vi "LISVwithout21-10-2019.vi"() -> ()   [LabVIEW 2018]
uses:
  <instrlib>/Keithley 6517/Keithley 6517.lvlib
  <instrlib>/Keithley 2450/Keithley 2450.lvlib
panel:
  out "Photodiode":cluster{dbl[], dbl[]}(graph)
  out "LED":cluster{dbl[], dbl[]}(graph)
  out "Number of times the K6514 buffer wait loop ran":i32
  in  "Measure settings":T1={"Keithley 2450 \nMeasurement speed (PLC)"=1.0, "High capacitance?"=FALSE, "Keithley 6514 \nMeasurement speed (PLC)"=0.05, "LED: number of readings to average/measurement"=10, "Photodiode: number of readings to average/measurement"=10, "OD3 engaged on 918D?"=TRUE} {"Photodiode: number of readings to average/measurement" items=["10"=10, "50"=50, "100"=100]; "LED: number of readings to average/measurement" items=["10"=10, "50"=50, "100"=100]}
  out "Number of Readings Retrieved from K6514":i32
  in  "File I/O (in strings below, use a single word, no spaces or special characters other than -)":T2={"Experiment Name"="", "LV Data folder"=path "", "Device number"=1, "Repetition Number"=1, "Extra comment"=""}
  in  "LED bias settings":T3={"Steps (number)"=51, "Vdevice (starting, V)"=0.0, "Vdevice (ending, V)"=5.0, "Accurate readback?"=TRUE, "Current compliance (A)"=0.1} {"Vdevice (ending, V)" min=0.1 max=12.0 step=0.05; "Vdevice (starting, V)" min=0.0 max=20.0 step=0.05; "Steps (number)" min=5 max=1001 step=1}
  in  "VISA Resource IDs":T4={"VISA resource name (Keithley 2450)"="TCPIP0::192.168.30.14::inst0::INSTR", "VISA resource name (Keithley 6514)"="GPIB0::16::INSTR"}
  out "error out":errorcluster
  in  "error in (no error)":errorcluster
  # "1"
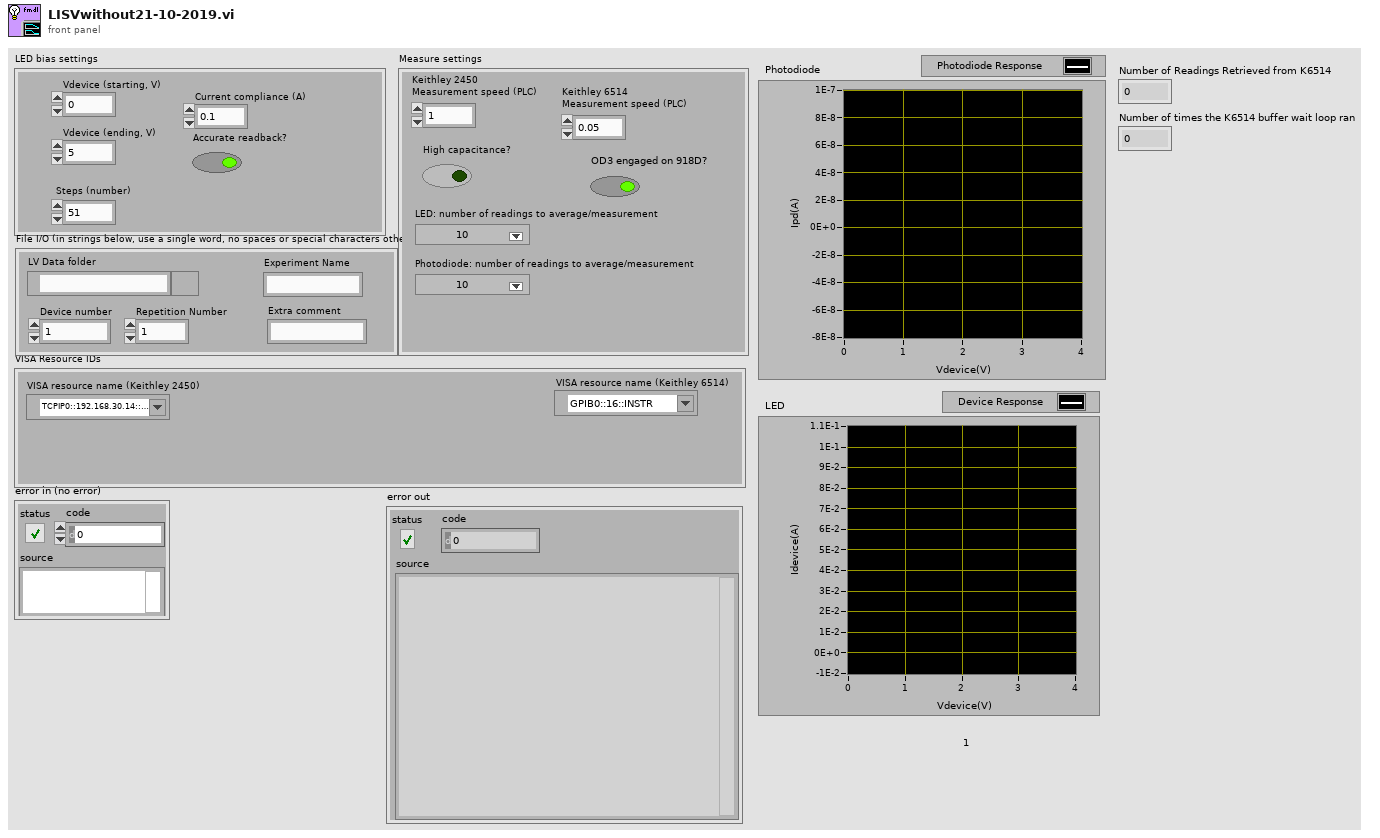
[diagram p1: front panel]
types:
  T1 = cluster{"Keithley 2450 \nMeasurement speed (PLC)":dbl, "High capacitance?":bool, "Keithley 6514 \nMeasurement speed (PLC)":dbl, "LED: number of readings to average/measurement":u16, "Photodiode: number of readings to average/measurement":u16, "OD3 engaged on 918D?":bool}
  T2 = cluster{"Experiment Name":string, "LV Data folder":path, "Device number":u32, "Repetition Number":u32, "Extra comment":string}
  T3 = cluster{"Steps (number)":i32, "Vdevice (starting, V)":dbl, "Vdevice (ending, V)":dbl, "Accurate readback?":bool, "Current compliance (A)":dbl}
  T4 = cluster{"VISA resource name (Keithley 2450)":refnum<visa-resource-name>, "VISA resource name (Keithley 6514)":refnum<visa-resource-name>}
  T5 = enum16{"open", "replace", "create", "open or create", "replace or create", "replace or create with confirmation"}
  T6 = cluster{dbl, "Mean":dbl, "StDev":dbl, "Mean":dbl, "Standard Deviation":dbl, dbl, dbl}
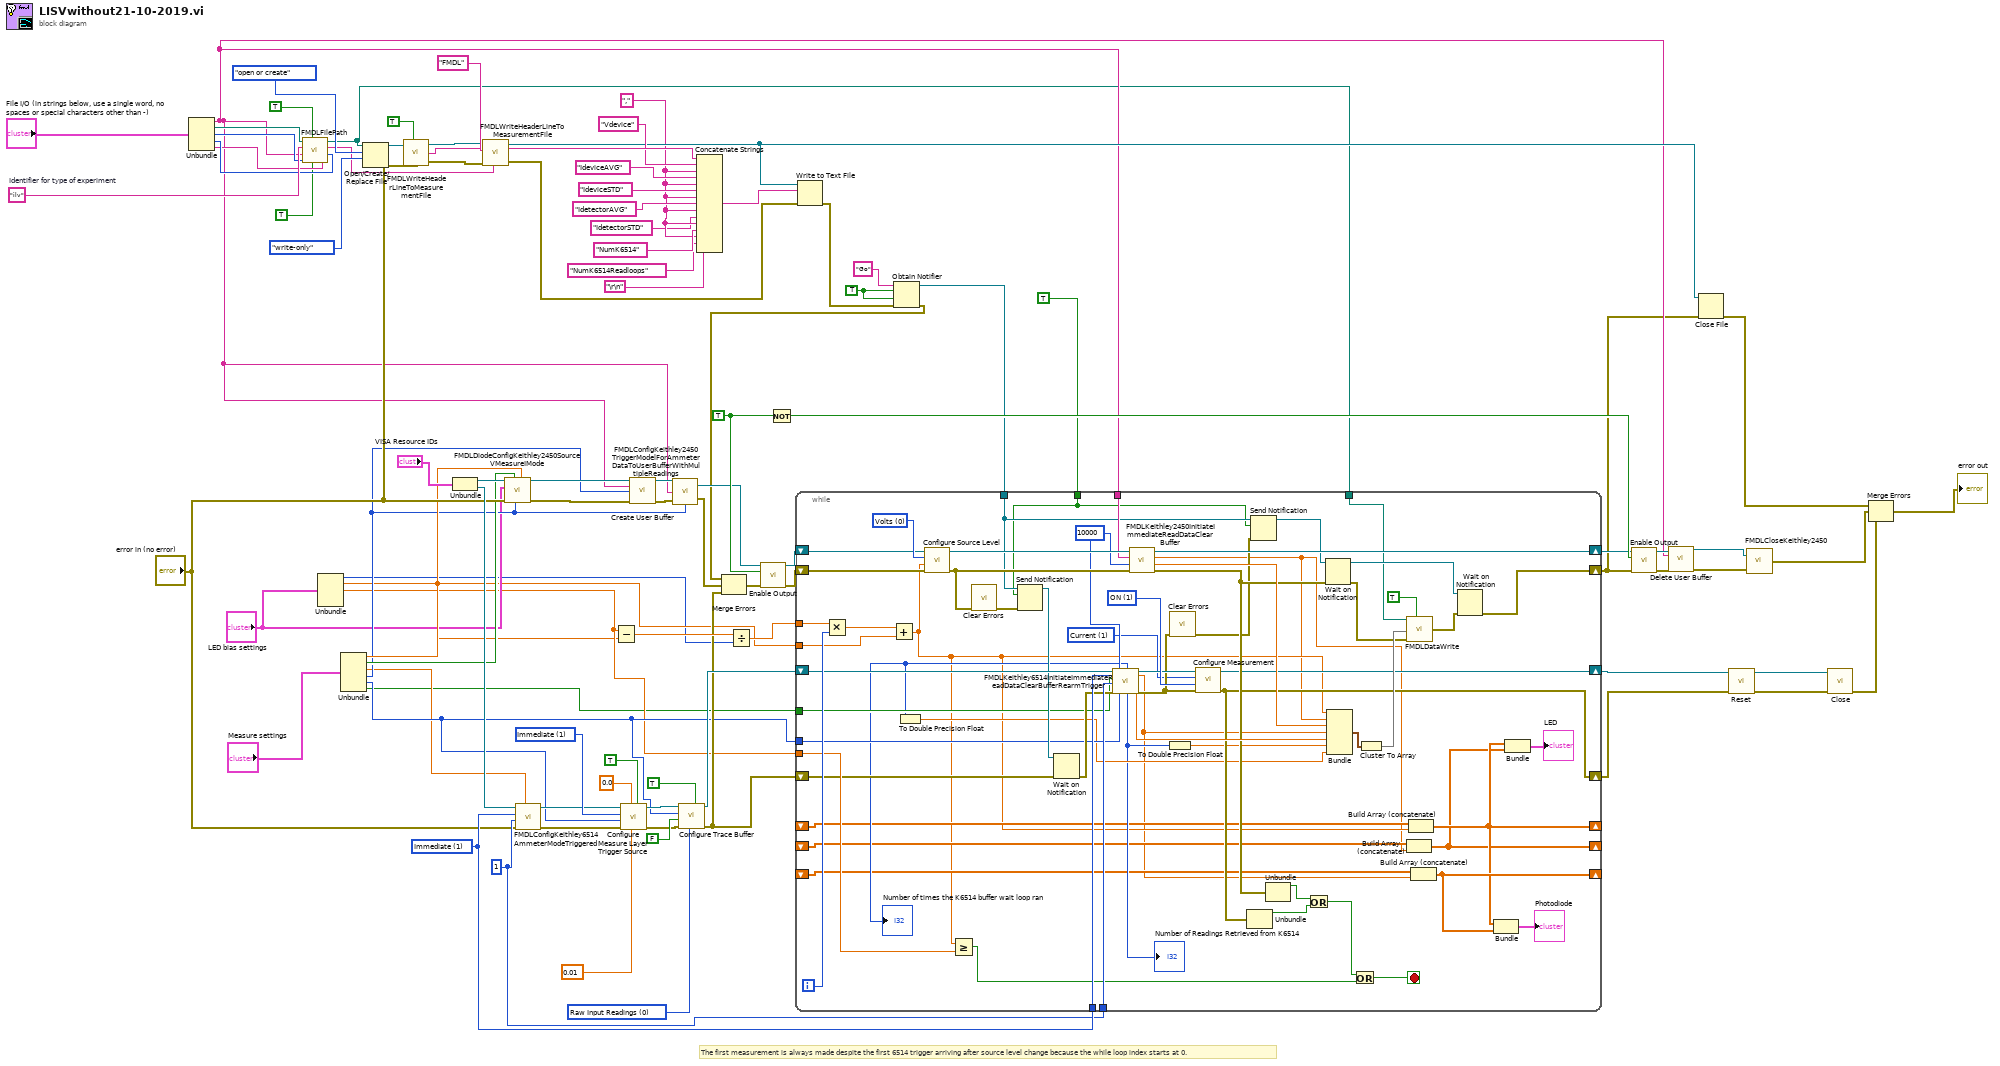
[diagram p0: block diagram]
diagram:
  w25 = TRUE ("create if not found? (T)")
  w9 = ","
  w67 = "ilv"  # Identifier for type of experiment
  w76 = 1 items=["Hold"=0, "Immediate"=1, "Manual"=3, "Bus"=4, "Trigger Link"=5, "External Triggering"=6, "Timer "=7] ("Measure Source (1: Immediate)")
  w77 = 1 ("Arm Count (1)")
  w78 = 1 items=["Hold", "Immediate", "Real-time Clock", "Manual", "Bus", "Trigger Link", "External Triggering", "Timer", "STest", "PSTest", "NSTest", "BSTest"] ("Arm Source (1: Immediate)")
  w81 = u16 0 items=["Raw Input Readings", "CALC1 Readings", "CALC2 Readings"] ("Buffer Source (0: Raw Input Readings)")
  w90 = TRUE ("Enable Output (T: Enable)")
  # "The first measurement is always made despite the first 6514 trigger arriving after source level change because the while loop index starts at 0."
  n1 = Unbundle("File I/O (in strings below, use a single word, no spaces or special characters other than -)") -> ("Experiment Name"=w36:string, "LV Data folder"=w68:path, "Device number"=w66:u32, "Repetition Number"=w65:u32, "Extra comment"=w64:string)
  n2 = call "FMDLFilePath.vi"("Extra comment"=w64, "Repetition Number"=w65, "Include seconds string?"=TRUE, "Include Year Month string?"=TRUE, "Experiment number"=w66, "Experiment Name"=w36, "Experiment Type"=w67, "Data folder"=w68) -> ("date/time string"=w52:string, "Unique Filepath"=w23:path)
  n3 = Unbundle("LED bias settings") -> ("Steps (number)"=w13:i32, "Vdevice (starting, V)"=w14:dbl, "Vdevice (ending, V)"=w15:dbl)  [unwired: 2 out]
  n4 = Unbundle("Measure settings") -> ("Keithley 2450 \nMeasurement speed (PLC)"=w20:dbl, "High capacitance?"=w19:bool, "Keithley 6514 \nMeasurement speed (PLC)"=w12:dbl, "LED: number of readings to average/measurement"=w17:u16, "Photodiode: number of readings to average/measurement"=w18:u16, "OD3 engaged on 918D?"=w11:bool)
  n5 = Open/Create/Replace File(file path (use dialog)=w23, error in="error in (no error)", operation (0:open)=T5."open or create", access (0:read/write)=enum16{"read/write", "read-only", "write-only"}."write-only") -> (refnum out=w57:refnum<file>, error out=w56:errorcluster)  [unwired: 2 in, 1 out]
  n6 = call "FMDLWriteHeaderLineToMeasurementFile.vi"("Refnum in"=w57, "Spacer Line?"=TRUE, "error in (no error)"=w56) -> ("refnum out"=w53:refnum<file>, "Comment character"=w51:string, "error out"=w55:errorcluster)  [unwired: 3 in]
  n7 = Unbundle ("unbundle2450,6514")("VISA Resource IDs") -> ("VISA resource name (Keithley 2450)"=w94:refnum<visa-resource-name>, "VISA resource name (Keithley 6514)"=w91:refnum<visa-resource-name>)
  n8 = call "FMDLWriteHeaderLineToMeasurementFile.vi"("Refnum in"=w53, "Header Key String"="FMDL", "Header Value String"=w52, "error in (no error)"=w55) -> ("refnum out"=w45:refnum<file>, "error out"=w31:errorcluster)  [unwired: 2 in, 1 out]
  n9 = call "FMDLDiodeConfigKeithley2450SourceVMeasureIMode.vi"("Measurement Speed (NPLC)"=w20, "Measurement Count"=w17, "Enable High Capacitance (T:Enable)"=w19, "error in (no error)"="error in (no error)", "LED bias settings"="LED bias settings", "VISA resource name in"=w94) -> ("error out"=w85:errorcluster, "VISA resource name out"=w86:refnum<visa-resource-name>)  [unwired: 4 in]
  n10 = call "FMDLConfigKeithley6514AmmeterModeTriggered.vi"("Integration Time (1 PLCs)"=w12, "error in (no error)"="error in (no error)", "Arm Count (1)"=w77, "Arm Source (1: Immediate)"=w78, "VISA resource name"=w91) -> ("error out"=w74:errorcluster, "VISA resource name out"=w75:refnum<visa-resource-name>)  [unwired: 5 in]
  n11 = Subtract(x=w15, y=w14) -> (x-y=w93:dbl)
  n12 = call <instrlib>:"Configure Measure Layer Trigger Source.vi"("Enable Auto Measure Delay (F: Disable)"=TRUE, "Measure Timer Interval (0.1)"=0.01, "Measure Delay (0 s)"=0.0, "error in (no error)"=w74, "Measure Count (1)"=w18, "Measure Source (1: Immediate)"=w76, "VISA resource name"=w75) -> ("error out"=w71:errorcluster, "VISA resource name out"=w70:refnum<visa-resource-name>)  [unwired: 3 in]
  n13 = call <instrlib>:"Create User Buffer.vi"("VISA resource name"=w86, "Buffer Name"=w36, "Buffer Size"=w17, "error in (no error)"=w85) -> ("VISA resource name out"=w43:refnum<visa-resource-name>, "error out"=w41:errorcluster)  [unwired: 10 in]
  n14 = call "FMDLConfigKeithley2450TriggerModelForAmmeterDataToUserBufferWithMultipleReadings.vi"("Trigger Count (1)"=w17, "error in (no error)"=w41, "Buffer Name (defbuffer1)"=w36, "VISA resource name"=w43) -> ("error out"=w27:errorcluster, "VISA resource name out"=w42:refnum<visa-resource-name>)
  n15 = call <instrlib>:"Configure Trace Buffer.vi"("Enable Buffer (0: Disable)"=TRUE, "Buffer Source (0: Raw Input Readings)"=w81, "error in (no error)"=w71, "Enable Auto Buffer Sizing (F: Disable)"=FALSE, "Buffer Size (100)"=w18, "VISA resource name"=w70) -> ("error out"=w28:errorcluster, "VISA resource name out"=w79:refnum<visa-resource-name>)  [unwired: 4 in]
  n16 = Concatenate Strings(w51, "Vdevice", w9, "IdeviceAVG", w9, "IdeviceSTD", w9, "IdetectorAVG", w9, "IdetectorSTD", w9, "NumK6514", w9, "NumK6514Readloops", "\r\n") -> (w46:string)
  n17 = Divide(x=w93, y=w13) -> (x/y=w92:dbl)
  n18 = Not(x=w90) -> (.not. x?=w89:bool)
  n19 = Write to Text File(file (use dialog)=w45, text=w46, error in=w31) -> (error out=w30:errorcluster)  [unwired: 1 in, 2 out]
  n20 = Obtain Notifier(name (unnamed)="Go", notification data type=w25, create if not found? (T)=w25, error in (no error)=w30) -> (notifier out=w32:refnum<notifier>, error out=w26:errorcluster)  [unwired: 1 out]
  n21 = Merge Errors(w26, w27, w28) -> (w80:errorcluster)
  n22 = call <instrlib>:"Enable Output.vi"("error in (no error)"=w80, "Enable Output (T: Enable)"=w90, "VISA resource name"=w42) -> ("error out"=w87:errorcluster, "VISA resource name out"=w88:refnum<visa-resource-name>)  [unwired: 7 in]
  n23 = while {
    tunnel: w92 -> [w157]
    tunnel: w14 -> [w156]
    tunnel: w15 -> [w154]
    tunnel: w36 -> [w140]
    shift-right: [w120] -> w22
    shift-left: w87 -> [w151]
    shift-right: [w139] -> w84
    shift-left: w88 -> [w152]
    shift-right: [w115] -> w4
    shift-left: w79 -> [w150]
    tunnel: w78 -> [w147]
    tunnel: w77 -> [w149]
    tunnel: w32 -> [w129]
    tunnel: TRUE -> [w128]
    tunnel: w18 -> [w127]
    tunnel: w23 -> [w123]
    tunnel: w11 -> [w118]
    shift-right: [w113] -> w2
    shift-left: w28 -> [w145]
    shift-right: [w101] -> _
    shift-left: _ -> [w106]
    shift-right: [w100] -> _
    shift-left: _ -> [w105]
    shift-right: [w103] -> _
    shift-left: _ -> [w104]
    i -> [w158]
    stop <- w135 stop-if-true
    w112 = 1 items=["Voltage", "Current", "Resistance", "Charge"] ("Measurement Function (0: Voltage)")
    w117 = 1 items=["OFF", "ON", "ONCE"] ("Auto Range (1: ON)")
    w119 = u32 10000 ("Timeout (10000 ms)")
    w153 = u16 0 items=["Volts", "Current"] ("Function (0: Volts)")
    n24 = Multiply(x=w157, y=w158) -> (x*y=w155:dbl)
    n25 = Add(x=w155, y=w156) -> (x+y=w98:dbl)
    n26 = call <instrlib>:"Configure Source Level.vi"("error in (no error)"=w151, "Source Level (1.0)"=w98, "Function (0: Volts)"=w153, "VISA resource name"=w152) -> ("error out"=w141:errorcluster, "VISA resource name out"=w142:refnum<visa-resource-name>)  [unwired: 6 in]
    n27 = Greater Or Equal?(x=w98, y=w154) -> (x >= y?=w136:bool)
    n28 = call <vilib>:"Clear Errors.vi"("error in (no error)"=w141) -> ("error out"=w146:errorcluster)  [unwired: 5 in, 1 out]
    n29 = Send Notification(notification=w128, notifier=w129, error in (no error)=w146) -> (notifier out=w144:refnum<notifier>)  [unwired: 1 out]
    n30 = Wait on Notification(notifier=w144, error in (no error)=w145) -> (error out=w143:errorcluster)  [unwired: 2 in, 3 out]
    n31 = call "FMDLKeithley6514InitiateImmediateReadDataClearBufferRearmTrigger.vi"("VISA resource name"=w150, "Arm Source (1: Immediate)"=w147, "OD3 engaged on 918D?"=w118, "Arm Count (1)"=w149, "error in (no error)"=w143, "Timeout (10000 ms)"=w119, "Buffer size previously set"=w127) -> ("Number of times the loop ran"=w109:i32, "Number of Readings in K6514 Buffer"=w108:i32, "VISA resource name out"=w116:refnum<visa-resource-name>, "Mean"=w96:dbl, "Standard Deviation"=w148:dbl, "error out"=w114:errorcluster)  [unwired: 4 in, 3 out]
    "Number of Readings Retrieved from K6514" <- w108
    "Number of times the K6514 buffer wait loop ran" <- w109
    n32 = To Double Precision Float(number=w109) -> (double precision float=w110:dbl)
    n33 = call "FMDLKeithley2450InitiateImmediateReadDataClearBuffer.vi"("error in (no error)"=w141, "Timeout (10000 ms)"=w119, "Buffer Name (defbuffer1)"=w140, "VISA resource name"=w142) -> ("error out"=w132:errorcluster, "StDev"=w138:dbl, "Mean"=w97:dbl, "VISA resource name out"=w139:refnum<visa-resource-name>)  [unwired: 3 out]
    n34 = To Double Precision Float(number=w108) -> (double precision float=w107:dbl)
    n35 = call <vilib>:"Clear Errors.vi"("error in (no error)"=w114) -> ("error out"=w131:errorcluster)  [unwired: 5 in, 1 out]
    n36 = call <instrlib>:"Configure Measurement.vi"("error in (no error)"=w114, "Auto Range (1: ON)"=w117, "Measurement Function (0: Voltage)"=w112, "VISA resource name"=w116) -> ("error out"=w113:errorcluster, "VISA resource name out"=w115:refnum<visa-resource-name>)  [unwired: 6 in]
    n37 = Unbundle(w113) -> ("status"=w134:bool)  [unwired: 2 out]
    n38 = Send Notification(notification=w128, notifier=w129, error in (no error)=w131) -> (notifier out=w130:refnum<notifier>)  [unwired: 1 out]
    n39 = Unbundle(w132) -> ("status"=w133:bool)  [unwired: 2 out]
    n40 = Or(x=w133, y=w134) -> (x .or. y?=w137:bool)
    n41 = Wait on Notification(notifier=w130, error in (no error)=w132) -> (notifier out=w126:refnum<notifier>, error out=w124:errorcluster)  [unwired: 2 in, 2 out]
    n42 = Bundle(w98, "Mean"=w97, "StDev"=w138, "Mean"=w96, "Standard Deviation"=w148, w107, w110) -> (w111:T6)  [unwired: 1 in]
    n43 = Or(x=w137, y=w136) -> (x .or. y?=w135:bool)
    n44 = Cluster To Array(cluster=w111) -> (array=w125:dbl[])
    n45 = Build Array (concatenate)(w105, w97) -> (w100:dbl[])
    n46 = call "FMDLDataWrite.vi"("append to file? (new file:F)"=TRUE, "error in (no error)"=w124, "1D data"=w125, "file path (dialog if empty)"=w123) -> ("error out"=w121:errorcluster)  [unwired: 2 in]
    n47 = Build Array (concatenate)(w106, w98) -> (w101:dbl[])
    n48 = Build Array (concatenate)(w104, w96) -> (w103:dbl[])
    n49 = Wait on Notification(notifier=w126, error in (no error)=w121) -> (error out=w120:errorcluster)  [unwired: 2 in, 3 out]
    n50 = Bundle(w101, w103) -> (→"Photodiode":cluster{dbl[], dbl[]})  [unwired: 1 in]
    n51 = Bundle(w101, w100) -> (→"LED":cluster{dbl[], dbl[]})  [unwired: 1 in]
  }
  n52 = call <instrlib>:"Enable Output.vi"("error in (no error)"=w22, "Enable Output (T: Enable)"=w89, "VISA resource name"=w84) -> ("error out"=w39:errorcluster, "VISA resource name out"=w40:refnum<visa-resource-name>)  [unwired: 7 in]
  n53 = call <instrlib>:"Delete User Buffer.vi"("VISA resource name"=w40, "Buffer Name (defbuffer1)"=w36, "error in (no error)"=w39) -> ("VISA resource name out"=w38:refnum<visa-resource-name>, "error out"=w37:errorcluster)  [unwired: 11 in]
  n54 = Close File(refnum=w45, error in=w22) -> (error out=w44:errorcluster)  [unwired: 1 out]
  n55 = call <instrlib>:"Reset.vi"("error in (no error)"=w2, "VISA resource name"=w4) -> ("error out"=w5:errorcluster, "VISA resource name out"=w3:refnum<visa-resource-name>)  [unwired: 8 in]
  n56 = call "FMDLCloseKeithley2450.vi"("error in (no error)"=w37, "VISA resource name"=w38) -> ("error out"=w34:errorcluster)
  n57 = call <instrlib>:"Close.vi"("error in (no error)"=w5, "VISA resource name"=w3) -> ("error out"=w33:errorcluster)  [unwired: 9 in]
  n58 = Merge Errors(w44, w34, w33) -> (→"error out":errorcluster)
